vi "Separate 4ROI_new.vi"(0 "ROI Descriptor":T1 {"Contours"."Type" items=["No Selection", "Point", "Line", "Rectangle", "Oval", "Polygon", "Freehand Region", "Annulus", "Unused2", "Unused3", "Broken Line", "Freehand Line", "Rotated Rectangle"]}, 5 "ROIsize":cluster{"Width":dbl, "Height":dbl}[](array[cluster]), 11 "error in":errorcluster) -> (4 "Left ROI":T1 {"Contours"."Type" items=["No Selection", "Point", "Line", "Rectangle", "Oval", "Polygon", "Freehand Region", "Annulus", "Unused2", "Unused3", "Broken Line", "Freehand Line", "Rotated Rectangle"]}, 6 "Top ROI":T1 {"Contours"."Type" items=["No Selection", "Point", "Line", "Rectangle", "Oval", "Polygon", "Freehand Region", "Annulus", "Unused2", "Unused3", "Broken Line", "Freehand Line", "Rotated Rectangle"]}, 8 "Right ROI":T1 {"Contours"."Type" items=["No Selection", "Point", "Line", "Rectangle", "Oval", "Polygon", "Freehand Region", "Annulus", "Unused2", "Unused3", "Broken Line", "Freehand Line", "Rotated Rectangle"]}, 10 "Bottom ROI":T1 {"Contours"."Type" items=["No Selection", "Point", "Line", "Rectangle", "Oval", "Polygon", "Freehand Region", "Annulus", "Unused2", "Unused3", "Broken Line", "Freehand Line", "Rotated Rectangle"]}, 15 "error out":errorcluster)   [LabVIEW 2015]
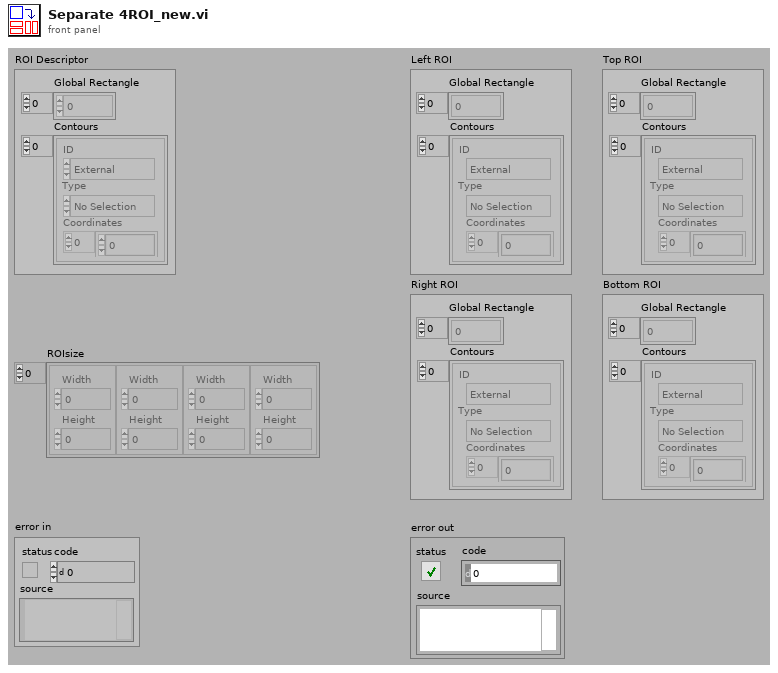
[diagram p1: front panel]
types:
  T1 = typedef "ROI Descriptor" = cluster{"Global Rectangle":i32[], "Contours":cluster{"ID":enum32{"External", "Internal"}, "Type":u32, "Coordinates":i32[]}[]}
  T2 = typedef "IMAQ Rectangle" = cluster{"Left":i32, "Top":i32, "Right":i32, "Bottom":i32, "Rotation":dbl}
  T3 = typedef "IMAQ Point" = cluster{"X":sgl, "Y":sgl}
  T4 = cluster{"MiddleRight_X":dbl, "MiddleRight_Y":dbl}
  T5 = cluster{"MiddleBottom_X":dbl, "MiddleBottom_Y":dbl}
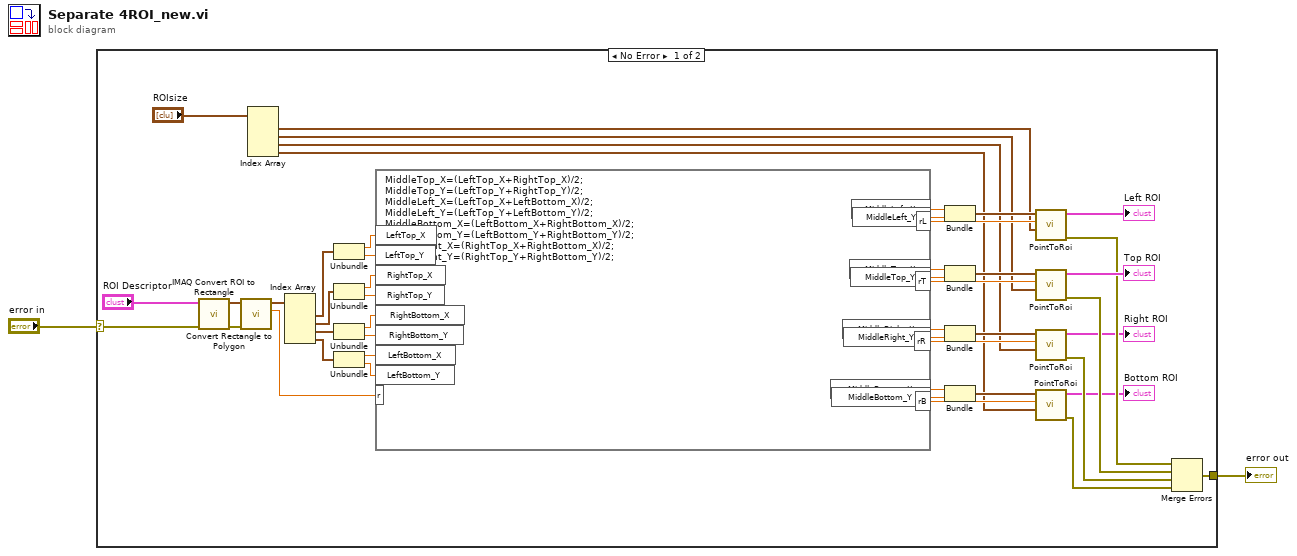
[diagram p0: block diagram]
diagram:
  n1 = case shown="No Error" "error in" {
    selector: "error in" -> [w5 w51]
    tunnel: [w10 w51] -> w2
    frame No Error {
      n2 = call "IMAQ Convert ROI to Rectangle"("error in (no error)"=w5, "ROI Descriptor"="ROI Descriptor") -> ("error out"=w19:errorcluster, "Rectangle"=w22:T2)  [unwired: 7 in]
      n3 = call "Convert Rectangle to Polygon.vi"("error in (no error)"=w19, "Rectangle"=w22) -> ("Rotation"=w20:dbl, "Rectangle Points"=w21:T3[])  [unwired: 7 in, 1 out]
      n4 = Index Array(array="ROIsize") -> (element #1=w9:cluster{"Width":dbl, "Height":dbl}, element #2=w8:cluster{"Width":dbl, "Height":dbl}, element #3=w7:cluster{"Width":dbl, "Height":dbl}, element #4=w6:cluster{"Width":dbl, "Height":dbl})  [unwired: 4 in]
      n5 = Index Array(array=w21) -> (element #1=w29:T3, element #2=w28:T3, element #3=w50:T3, element #4=w30:T3)  [unwired: 4 in]
      n6 = Unbundle(w29) -> ("X"=w49:sgl, "Y"=w48:sgl)
      n7 = Unbundle(w28) -> ("X"=w47:sgl, "Y"=w46:sgl)
      n8 = Unbundle(w50) -> ("X"=w45:sgl, "Y"=w44:sgl)
      n9 = Unbundle(w30) -> ("X"=w43:sgl, "Y"=w42:sgl)
      n10 = formula code="MiddleTop_X=(LeftTop_X+RightTop_X)/2;\nMiddleTop_Y=(LeftTop_Y+RightTop_Y)/2;\nMiddleLeft_X=(LeftTop_X+LeftBottom_X)/2;\nMiddleLeft_Y=(LeftTop_Y+LeftBottom_Y)/2;\nMiddleBottom_X=(LeftBottom_X+RightBottom_X)/2;\nMiddleBottom_Y=(LeftBottom_Y+RightBottom_Y)/2;\nMiddleRight_X=(RightTop_X+RightBottom_X)/2;\nMiddleRight_Y=(RightTop_Y+RightBottom_Y)/2;\nrT=r+0;\nrL=r+90;\nrB=r+180;\nrR=r+270;"("LeftTop_X"=w49, "LeftTop_Y"=w48, "RightTop_X"=w47, "RightTop_Y"=w46, "RightBottom_X"=w45, "RightBottom_Y"=w44, "LeftBottom_X"=w43, "LeftBottom_Y"=w42, "r"=w20) -> ("MiddleTop_X"=w41:dbl, "MiddleTop_Y"=w40:dbl, "MiddleLeft_X"=w39:dbl, "MiddleLeft_Y"=w38:dbl, "MiddleRight_X"=w37:dbl, "MiddleRight_Y"=w36:dbl, "MiddleBottom_X"=w35:dbl, "MiddleBottom_Y"=w34:dbl, "rT"=w23:dbl, "rL"=w24:dbl, "rR"=w25:dbl, "rB"=w26:dbl)
      n11 = Bundle("MiddleLeft_X"=w39, "MiddleLeft_Y"=w38) -> (w33:cluster{"MiddleLeft_X":dbl, "MiddleLeft_Y":dbl})  [unwired: 1 in]
      n12 = Bundle("MiddleTop_X"=w41, "MiddleTop_Y"=w40) -> (w18:cluster{"MiddleTop_X":dbl, "MiddleTop_Y":dbl})  [unwired: 1 in]
      n13 = Bundle("MiddleRight_X"=w37, "MiddleRight_Y"=w36) -> (w32:T4)  [unwired: 1 in]
      n14 = Bundle("MiddleBottom_X"=w35, "MiddleBottom_Y"=w34) -> (w31:T5)  [unwired: 1 in]
      n15 = call "PointToRoi.vi"("ROISize"=w9, "r"=w24, "Point"=w33) -> ("error out"=w14:errorcluster, "ROI Descriptor"=→"Left ROI":T1)  [unwired: 7 in]
      n16 = call "PointToRoi.vi"("ROISize"=w8, "r"=w23, "Point"=w18) -> ("error out"=w13:errorcluster, "ROI Descriptor"=→"Top ROI":T1)  [unwired: 7 in]
      n17 = call "PointToRoi.vi"("ROISize"=w7, "r"=w25, "Point"=w32) -> ("error out"=w12:errorcluster, "ROI Descriptor"=→"Right ROI":T1)  [unwired: 7 in]
      n18 = call "PointToRoi.vi"("ROISize"=w6, "r"=w26, "Point"=w31) -> ("error out"=w11:errorcluster, "ROI Descriptor"=→"Bottom ROI":T1)  [unwired: 7 in]
      n19 = Merge Errors(w14, w13, w12, w11) -> (w10:errorcluster)
    }
    frame Error {
    }
  }
  "error out" <- w2
